vi "PluginLoader Ping.vi"(6 "contextId":T1, 8 "error in":errorcluster, 9 "timeout (ms)":i32=-1, 10 "Request Data":T5, 11 "gRPC ID":T1) -> (0 "error out":errorcluster, 2 "Response Data":T2, 3 "gRPC ID out":T1)   [LabVIEW 2021, in "CIF_PluginLoader_client.lvlib"]
uses:
  CIF_PluginLoader_client.lvlib
  <vilib>/gRPC/LabVIEW gRPC Library/Shared/grpcId.ctl
  RPC Messages/cif_pluginloader_PingRequest.ctl
  RPC Messages/cif_pluginloader_PingResponse.ctl
  RPC Messages/cif_management_common_LoaderInfoFull.ctl
  RPC Messages/cif_management_common_LoaderType.ctl
  RPC Messages/cif_pluginloader_PingResponse_Flat.ctl
  RPC Messages/cif_management_common_LoaderInfoFull_Flat.ctl
  14035477-4c25-4107-8ed5-d0c4ef420ce5.vi
  <vilib>/gRPC/LabVIEW gRPC Library/Shared/TranslateGrpcError.vi
  <vilib>/gRPC/LabVIEW gRPC Library/Shared/Wait On Occurrence.vi
  RPC Messages/FlatToRichcif_management_common_LoaderInfoFull.vi
  <vilib>/gRPC/LabVIEW gRPC Library/Shared/Is Feature Enabled.vi
  <vilib>/gRPC/LabVIEW gRPC Library/Server API/Server/Get Server DLL Path.vi
  <vilib>/Utility/error.llb/Error Cluster From Error Code.vi
  <vilib>/gRPC/LabVIEW gRPC Library/grpc-lvsupport-release.lvlib
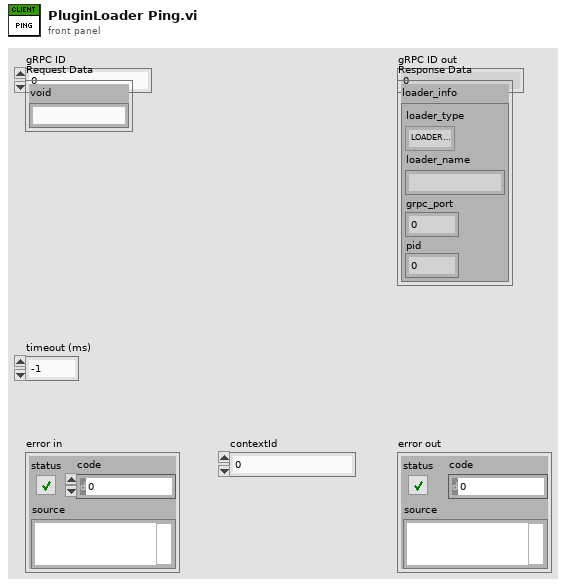
[diagram p1: front panel]
types:
  T1 = typedef "grpc-lvsupport-release.lvlib/grpcId.ctl" = u64
  T2 = typedef "CIF_PluginLoader_client.lvlib/cif_pluginloader_PingResponse.ctl" = cluster{"loader_info":T3}
  T3 = typedef "CIF_PluginLoader_client.lvlib/cif_management_common_LoaderInfoFull.ctl" = cluster{"loader_type":T4, "loader_name":string, "grpc_port":i32, "pid":u32}
  T4 = typedef "CIF_PluginLoader_client.lvlib/cif_management_common_LoaderType.ctl" = enum32{"LOADERTYPE_UNKNOWN", "LOADERTYPE_LABVIEW"}
  T5 = typedef "CIF_PluginLoader_client.lvlib/cif_pluginloader_PingRequest.ctl" = cluster{"void":string}
  T6 = typedef "CIF_PluginLoader_client.lvlib/cif_pluginloader_PingResponse_Flat.ctl" = cluster{"loader_info":T7}
  T7 = typedef "CIF_PluginLoader_client.lvlib/cif_management_common_LoaderInfoFull_Flat.ctl" = cluster{"loader_type":T4, "loader_name":string, "grpc_port":i32, "pid":u32}
  T8 = typedef "CIF_PluginLoader_client.lvlib/cif_pluginloader_PingRequest_Flat.ctl" = cluster{"void":string}
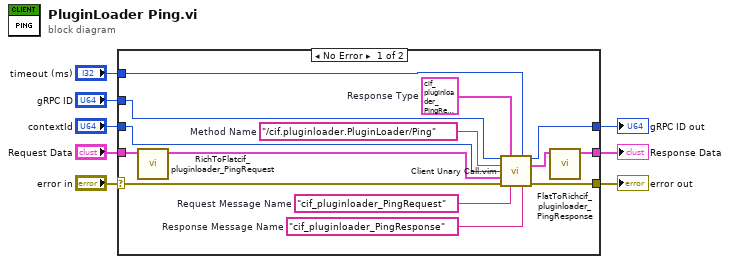
[diagram p0: block diagram]
diagram:
  n1 = case shown="No Error" "error in" {
    selector: "error in" -> [w18 w23]
    tunnel: [w17 w23] -> w7
    tunnel: "gRPC ID" -> [w16 w24]
    tunnel: [w15 w24] -> w5
    tunnel: "Request Data" -> [w12 _]
    tunnel: [w9 _] -> w3
    tunnel: "timeout (ms)" -> [w14 _]
    tunnel: "contextId" -> [w13 _]
    frame No Error {
      w19 = "cif_pluginloader_PingResponse"  # Response Message Name
      w20 = "cif_pluginloader_PingRequest"  # Request Message Name
      w21 = T6 {"loader_info"={"loader_type"=enum."LOADERTYPE_UNKNOWN", "loader_name"="", "grpc_port"=0, "pid"=0}}  # Response Type
      w22 = "/cif.pluginloader.PluginLoader/Ping"  # Method Name
      n2 = call "RichToFlatcif_pluginloader_PingRequest.vi"("InputCluster"=w12) -> ("OutputCluster"=w11:T8)  [unwired: 10 in]
      n3 = call "Client Unary Call.vim"("ClientID in"=w16, "Response Type"=w21, "timeout (ms)"=w14, "Method Name"=w22, "contextId"=w13, "Request Data"=w11, "error in"=w18, "Request Message Name"=w20, "Response Message Name"=w19) -> ("ClientID out"=w15:u64, "Response Data"=w10:T6, "error out"=w17:errorcluster)  [unwired: 4 in]
      n4 = call "FlatToRichcif_pluginloader_PingResponse.vi"("InputCluster"=w10) -> ("OutputCluster"=w9:T2)  [unwired: 10 in]
    }
    frame Error {
    }
  }
  "error out" <- w7
  "gRPC ID out" <- w5
  "Response Data" <- w3
